vi "ActionVIOnCompile.vi"(8 "error in (no error)":errorcluster, 11 "Device Item Ref in":T1 format="%.0x") -> (0 "error out":errorcluster)   [LabVIEW 2016, in "DDS Custom Device System Explorer.lvlib"]
uses:
  DDS Custom Device System Explorer.lvlib
  <vilib>/NI Veristand/Custom Device API/Custom Device Item Ref.ctl
  Shared/Compiled.Settings.ctl
  Shared/WriterReaderConfiguration.ctl
  Shared/Advanced DDS Configuration.ctl
  Shared/key Enum.ctl
  <vilib>/RTI DDS Toolkit/Types/RTI DDS ContentFilteredTopic Info.ctl
  Shared/Constants.vi
  <vilib>/NI Veristand/Custom Device Tools/Custom Device Utility Library/NI VeriStand - Search for All Items by GUID.vi
  <vilib>/NI Veristand/Custom Device API/Set Item Property (Variant).vi
  <vilib>/NI VeriStand/Custom Device API/Custom Device API.lvlib
  <vilib>/ni/NIVS Inline Async API/_Data Access System Explorer/Data Access System Explorer.lvlib
  <vilib>/NI VeriStand/Custom Device Tools/Custom Device Utility Library/Custom Device Utility Library.lvlib
  Shared/DDS Custom Device Shared.lvlib
  <vilib>/RTI DDS Toolkit/Library/LVDDS_library.lvlib
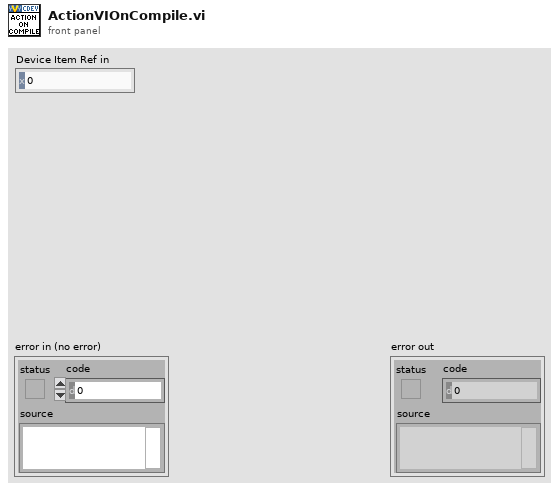
[diagram p1: front panel]
types:
  T1 = typedef "Custom Device API.lvlib/Custom Device Item Ref.ctl" = u64
  T2 = typedef "DDS Custom Device Shared.lvlib/Compiled.Settings.ctl" = cluster{"Name":string, "Topics":T3[]}
  T3 = typedef "DDS Custom Device Shared.lvlib/WriterReaderConfiguration.ctl" = cluster{"Topic Name":string, "Domain Id":u32, "Advanced Configuration":T4}
  T4 = typedef "DDS Custom Device Shared.lvlib/Advanced DDS Configuration.ctl" = cluster{"typeName":string, "key Name":T5, "domainParticipantQoSProfile":string, "dataWriterQoSProfile":string, "forceArrayMapping?":bool, "forceUnboundedString?":bool, "forceExclusiveReader?":bool, "forceRead? (only ExclusiveReader)":bool, "ContentFilteredTopic Info":T6}
  T5 = typedef "DDS Custom Device Shared.lvlib/key Enum.ctl" = enum16{"<none>", "I32_Num", "I64_Num", "U16_Num", "innercluster.Sgl_Num", "innercluster.Boolean"}
  T6 = typedef "LVDDS_library.lvlib/RTI DDS ContentFilteredTopic Info.ctl" = cluster{"Filter Type":string, "ContentFilteredTopic Name":string, "Filter Expression":string}
  T7 = enum16{"Output/Write", "Input/Read", "Input/ReadWrite"}
  T8 = cluster{"Name":string, "Type":enum16{"Output/Write", "Input/Read", "Input/ReadWrite"}, "VS Refs":T1[]}
  T9 = typedef "Custom Device API.lvlib/Custom Device Item Info.ctl" = cluster{"Name":string, "Is Channel":bool, "GUID":string, "Is Waveform":bool}
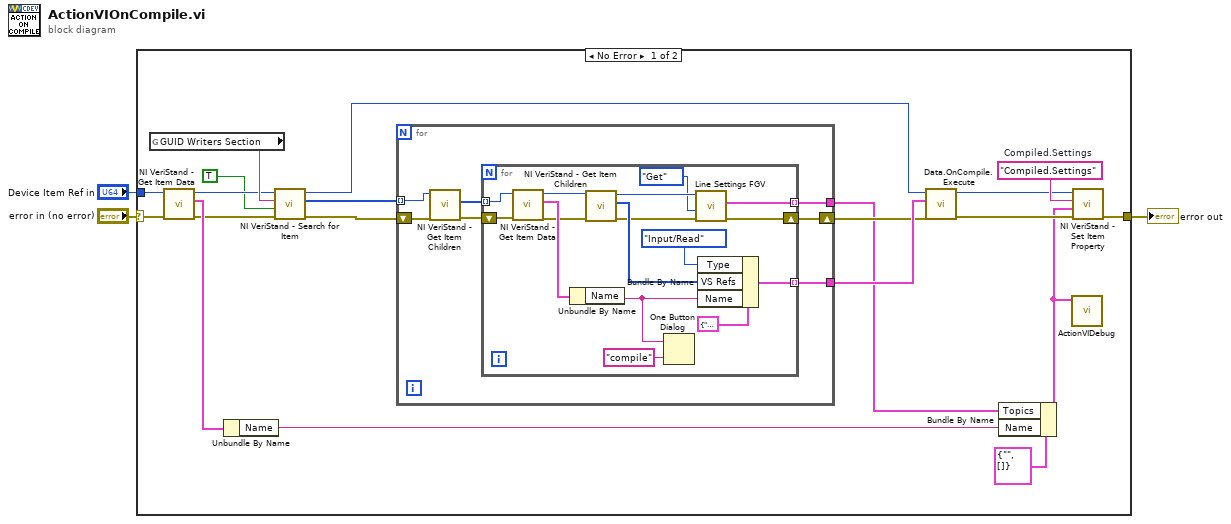
[diagram p0: block diagram]
diagram:
  n1 = case shown="No Error" "error in (no error)" {
    selector: "error in (no error)" -> [w21 w47]
    tunnel: [w22 w47] -> w2
    tunnel: "Device Item Ref in" -> [w20 _]
    frame No Error {
      w23 = "Compiled.Settings"  # Compiled.Settings
      n2 = global read "Constants.vi" "GUID Writers Section"() -> (w15:string)
      n3 = call <vilib>:"NI VeriStand - Get Item Data.vi"("error in (no error)"=w21, "Item Ref in"=w20) -> ("error out"=w14:errorcluster, "Item Info"=w19:T9, "Item Ref out"=w13:T1)  [unwired: 6 in, 1 out]
      n4 = Unbundle By Name(w19) -> ("Name"=w18:string)
      n5 = call-poly <vilib>:"NI VeriStand - Search for Item.vi"("error in"=w14, "Find All? (T)"=TRUE, "Item GUID"=w15, "Section Ref in"=w13) -> ("error out"=w11:errorcluster, "Item Refs"=w7:T1[], "Section Ref out"=w6:T1)  [unwired: 4 in, 1 out]
      n6 = for {
        tunnel: [w27] -> w10
        tunnel: [w25] -> w5
        shift-right: [w26] -> w9
        shift-left: w11 -> [w30]
        tunnel: w7 -> [w24] mode=indexing
        n7 = call <vilib>:"NI VeriStand - Get Item Children.vi"("error in (no error)"=w30, "Item Ref in"=w24) -> ("error out"=w28:errorcluster, "Child Refs"=w29:T1[])  [unwired: 6 in, 2 out]
        n8 = for {
          tunnel: w29 -> [w44] mode=indexing
          shift-right: [w36] -> w26
          shift-left: w28 -> [w43]
          tunnel: [w38] -> w27 mode=indexing
          tunnel: [w33] -> w25 mode=indexing
          n9 = call <vilib>:"NI VeriStand - Get Item Data.vi"("error in (no error)"=w43, "Item Ref in"=w44) -> ("error out"=w41:errorcluster, "Item Info"=w42:T9, "Item Ref out"=w40:T1)  [unwired: 6 in, 1 out]
          n10 = Unbundle By Name(w42) -> ("Name"=w32:string)
          n11 = call <vilib>:"NI VeriStand - Get Item Children.vi"("error in (no error)"=w41, "Item Ref in"=w40) -> ("error out"=w37:errorcluster, "Child Refs"=w39:T1[], "Item Ref out"=w35:T1)  [unwired: 6 in, 1 out]
          n12 = One Button Dialog(message=w32, button name ("OK")="compile") -> ()  [unwired: 1 out]
          n13 = call "Line Settings FGV.vi"("error in (no error)"=w37, "Get/Set"=enum16{"Set", "Get"}."Get", "Item Ref in"=w35) -> ("error out"=w36:errorcluster, "Line"=w33:T3)  [unwired: 6 in, 1 out]
          n14 = Bundle By Name(cluster=T8 {"Name"="", "Type"=enum."Output/Write", "VS Refs"=[]} ("Group"), "Type"=T7."Input/Read", "VS Refs"=w39, "Name"=w32) -> (w38:T8)
        }
      }
      n15 = call <vilib>:"Data.OnCompile.Execute.vi"("error in"=w9, "VS Ref Groups"=w10, "Custom Device Ref"=w6) -> ("error out"=w17:errorcluster, "Custom Device Ref"=w16:T1)  [unwired: 7 in]
      n16 = Bundle By Name(cluster=T2 {"Name"="", "Topics"=[]} ("Compiled.Settings"), "Topics"=w5, "Name"=w18) -> (w8:T2)
      n17 = call "ActionVIDebug.vi"("Compiled.Settings"=w8) -> ()  [unwired: 11 in]
      n18 = call-poly <vilib>:"NI VeriStand - Set Item Property.vi"("error in (no error)"=w17, "Value"=w8, "Property Name"=w23, "Item Ref in"=w16) -> ("error out"=w22:errorcluster)  [unwired: 5 in, 2 out]
    }
    frame Error {
    }
  }
  "error out" <- w2
